vi "View.vi"(8 "error out":errorcluster, 11 "2-Axis Stage":refnum<class "2-Axis Stage Async API.lvclass">) -> (0 "error out":errorcluster)   [LabVIEW 2022 SP3, in "View.lvlib"]
uses:
  View.lvlib
  Interfaces/2-Axis Stage API/2-Axis Stage Async API.lvclass
panel:
  out "XY Position Graph":cluster{"X":dbl, "Y":dbl}[](graph)
  in  "Abort Motion":bool
  in  "Home Stage":bool
  in  "Move Stage":bool
  in  "Y-Destination":dbl
  in  "X-Destination":dbl
  in  "Clear Error":bool
  out "Y-Speed":dbl
  in  "Set Y-Speed":u16
  in  "Set Y-Acceleration":u16
  out "Y-Current Speed":dbl
  out "Y-Acceleration":dbl
  out "Y-Homed":bool
  out "Y-Moving":bool
  out "Y-Position":dbl
  out "X-Speed":dbl
  in  "Set X-Speed":u16
  in  "Set X-Acceleration":u16
  out "X-Current Speed":dbl
  out "X-Acceleration":dbl
  out "X-Homed":bool
  out "X-Moving":bool
  out "X-Position":dbl
  out "Stage Error":errorcluster
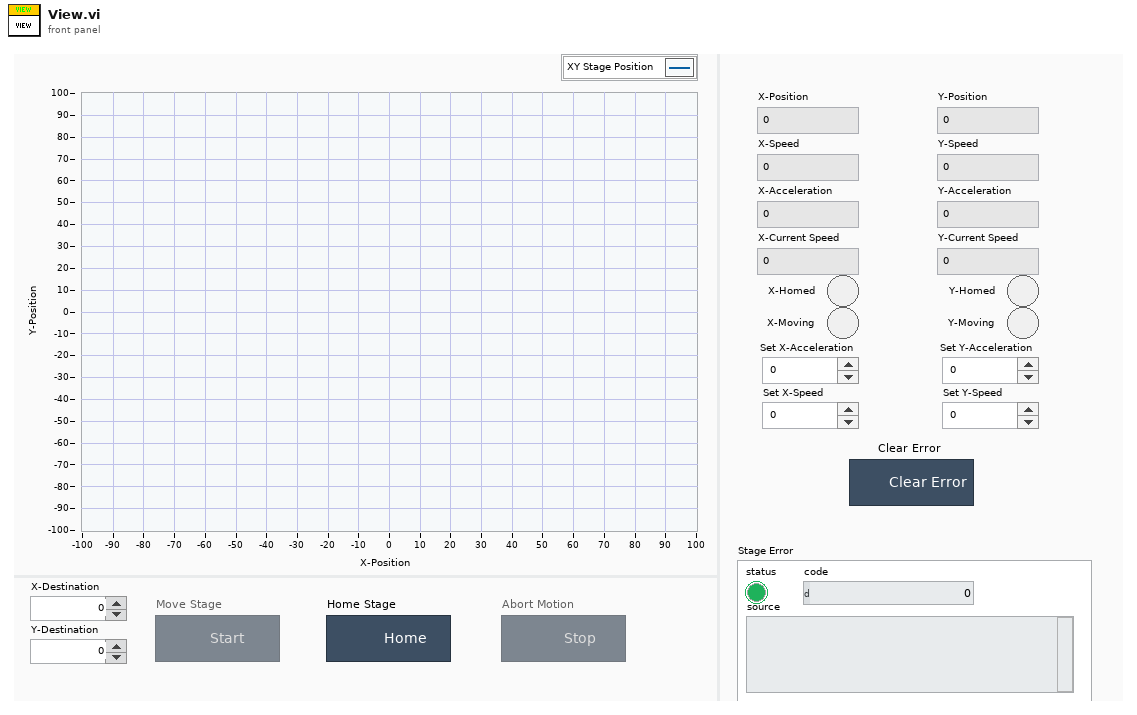
[diagram p1: front panel]
types:
  T1 = enum8{"Enabled", "Disabled", "Disabled and Grayed Out"}
  T2 = enum32{"Invalid", "Standard", "Closed", "Hidden", "Minimized", "Maximized"}
  T3 = enum32{"invalid app kind", "Development System", "Run Time System", "Student Edition", "Embedded LabVIEW", "Evaluation", "Custom"}
  T4 = cluster{"Current Position X":dbl, "Current Position Y":dbl}[]
  T5 = cluster{"Core":cluster{"Current VI Reference":refnum<vi>, "Close Panel on Exit?":bool}, "2-Axis Stage":refnum<class "2-Axis Stage Async API.lvclass">}
  T6 = cluster{"Current VI Reference":refnum<vi>, "Close Panel on Exit?":bool}
  T7 = cluster{"Event Registration Refnum":refnum<event-registration>, "Event Registration Refnum":refnum<event-registration>}
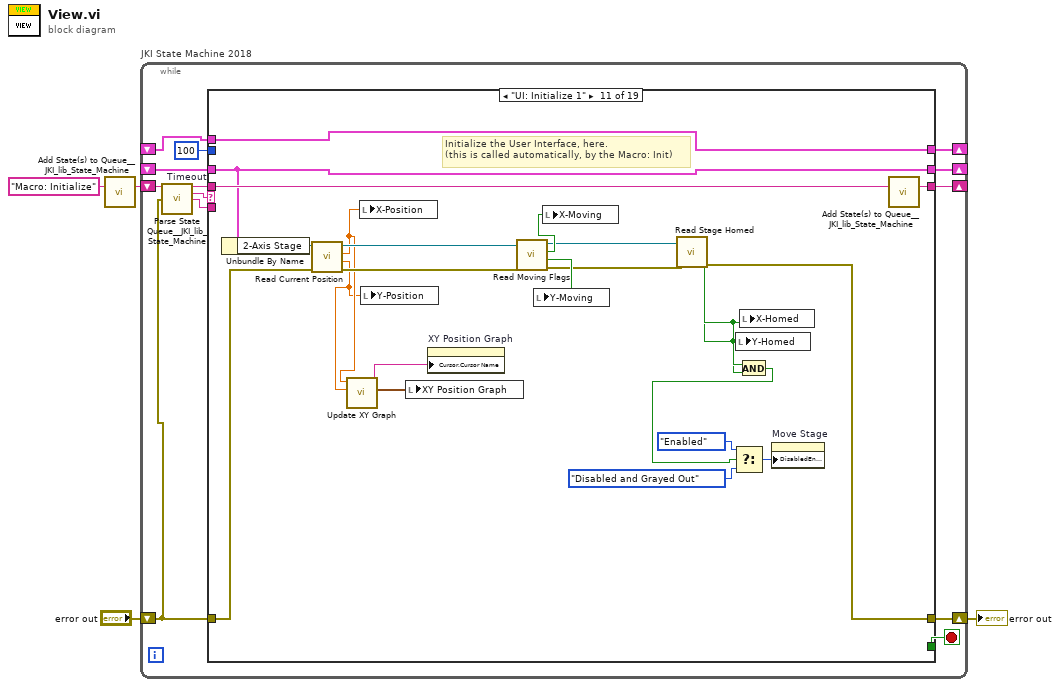
[diagram p0: block diagram]
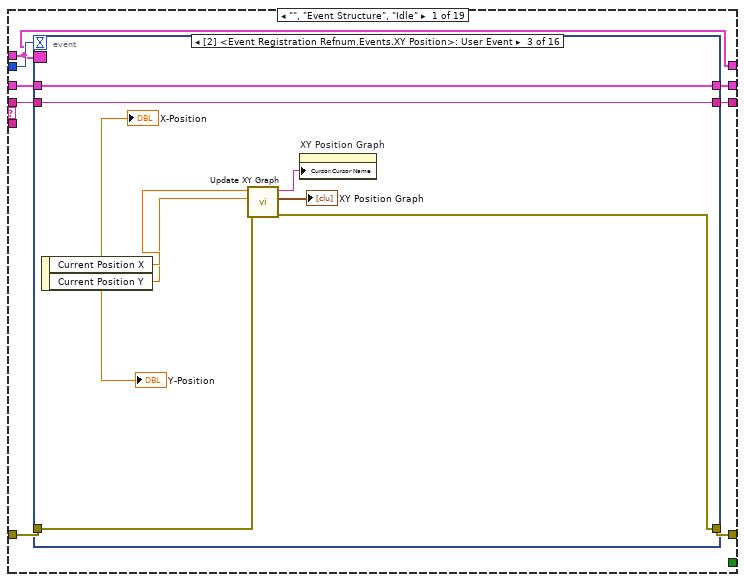
[diagram p2: hidden frame]
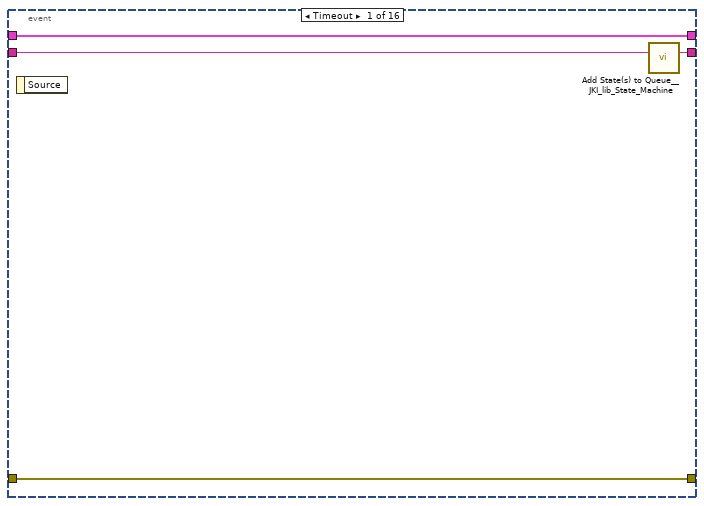
[diagram p3: hidden frame]
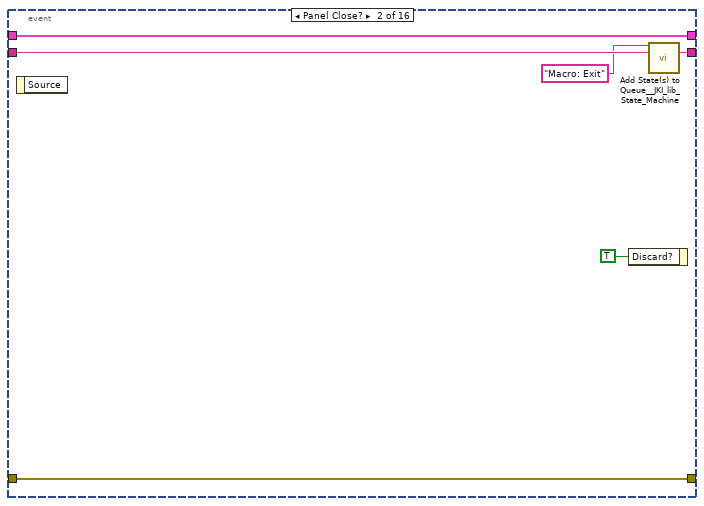
[diagram p4: hidden frame]
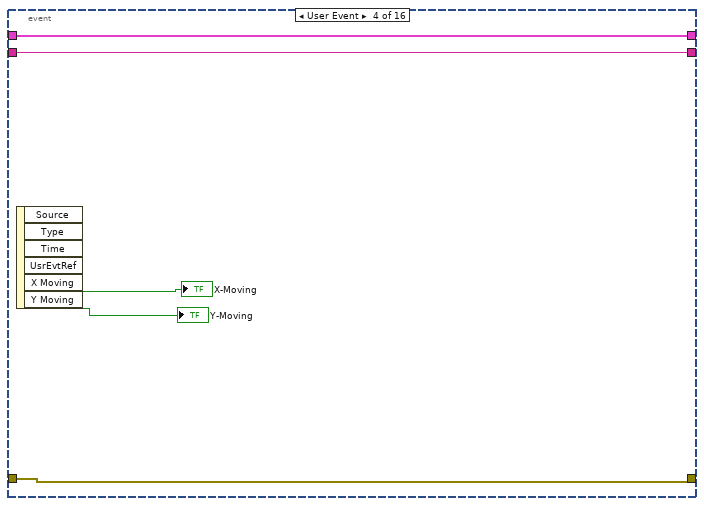
[diagram p5: hidden frame]
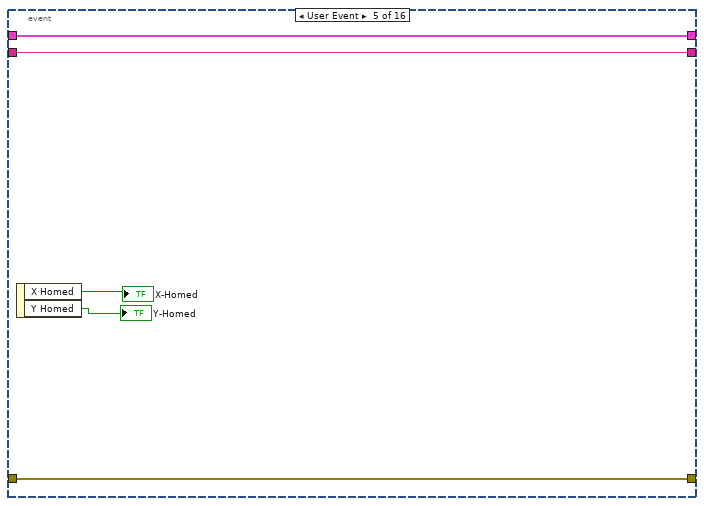
[diagram p6: hidden frame]
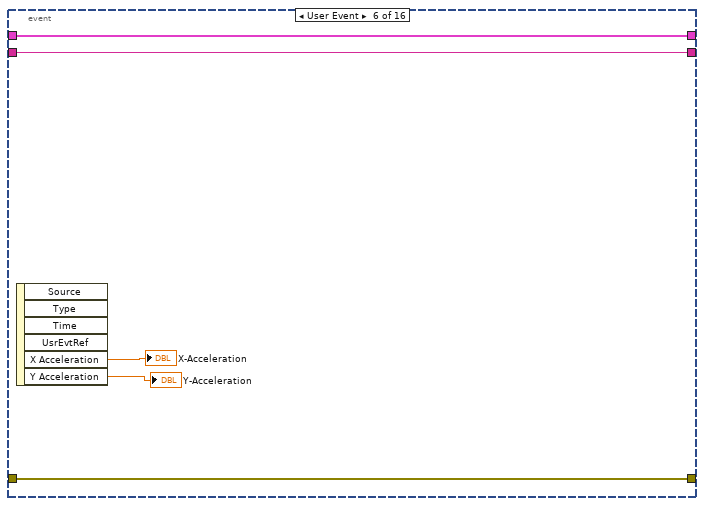
[diagram p7: hidden frame]
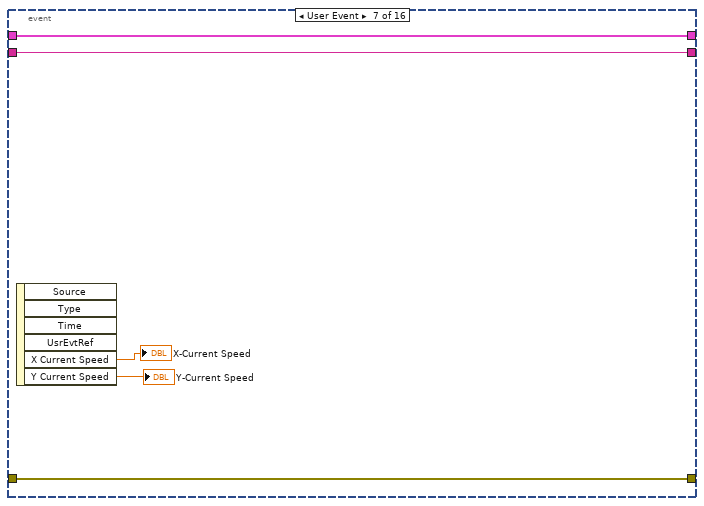
[diagram p8: hidden frame]
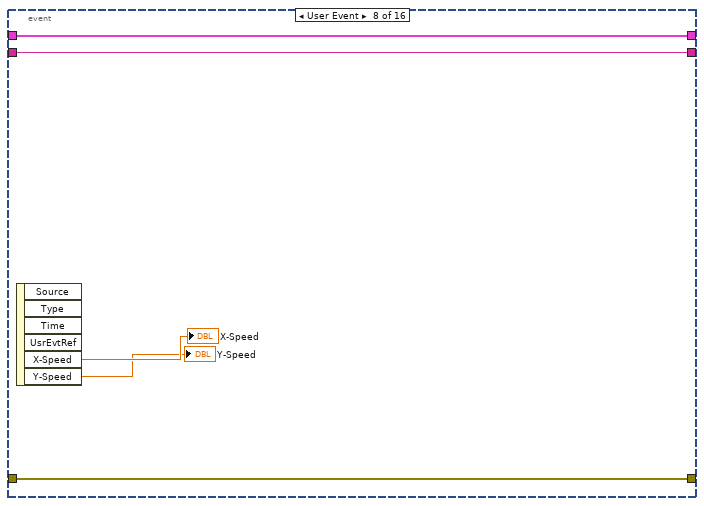
[diagram p9: hidden frame]
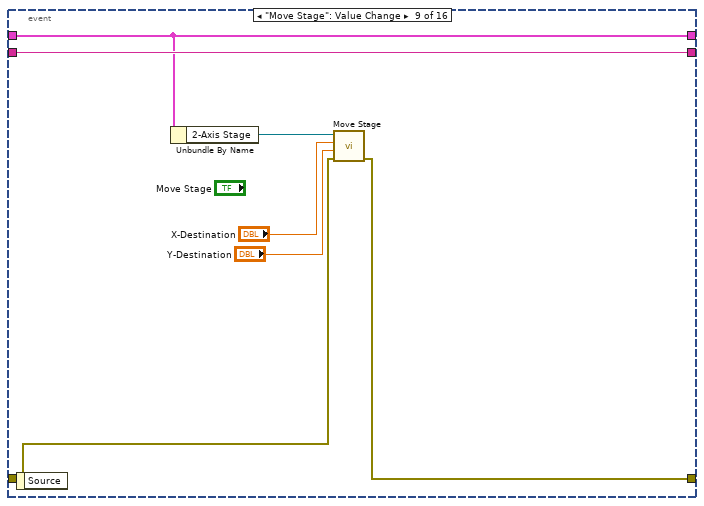
[diagram p10: hidden frame]
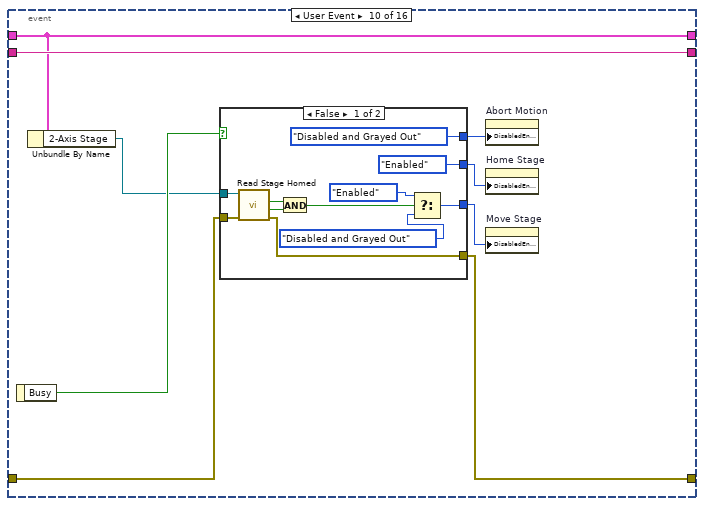
[diagram p11: hidden frame]
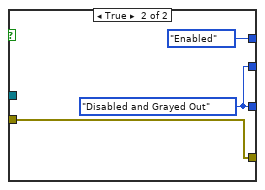
[diagram p12: hidden frame]
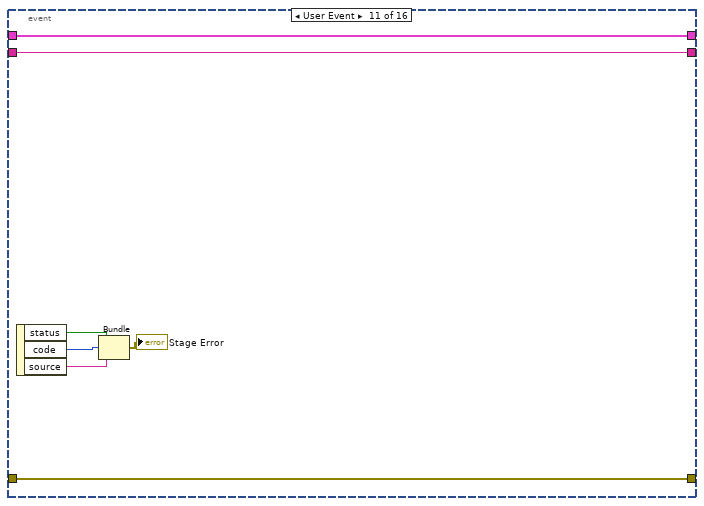
[diagram p13: hidden frame]
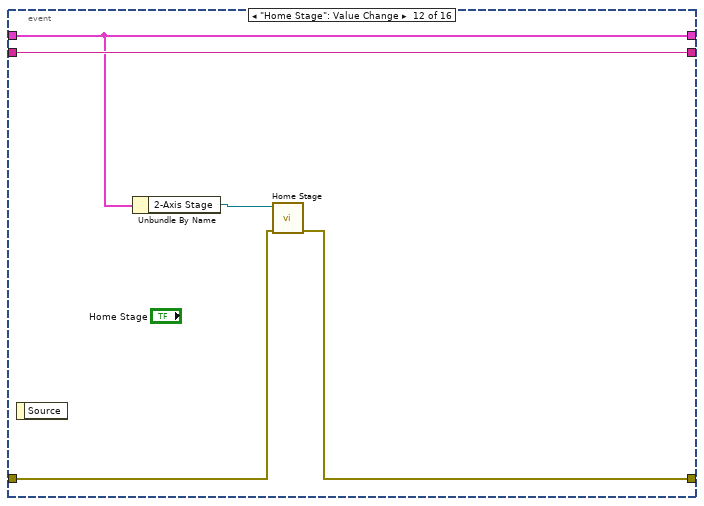
[diagram p14: hidden frame]
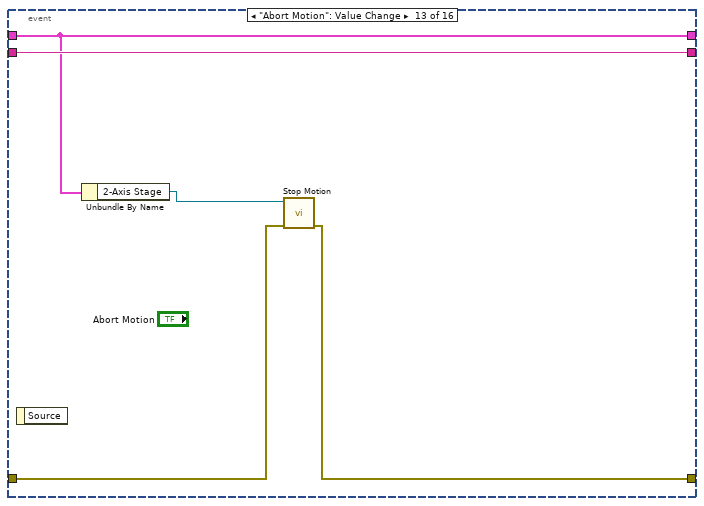
[diagram p15: hidden frame]
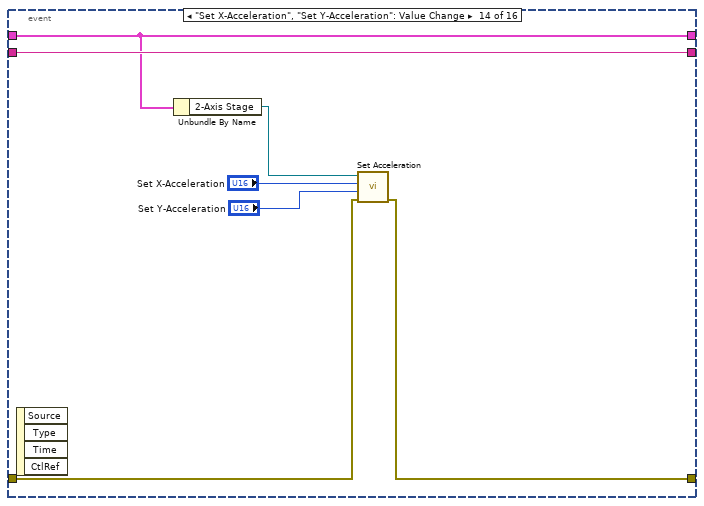
[diagram p16: hidden frame]
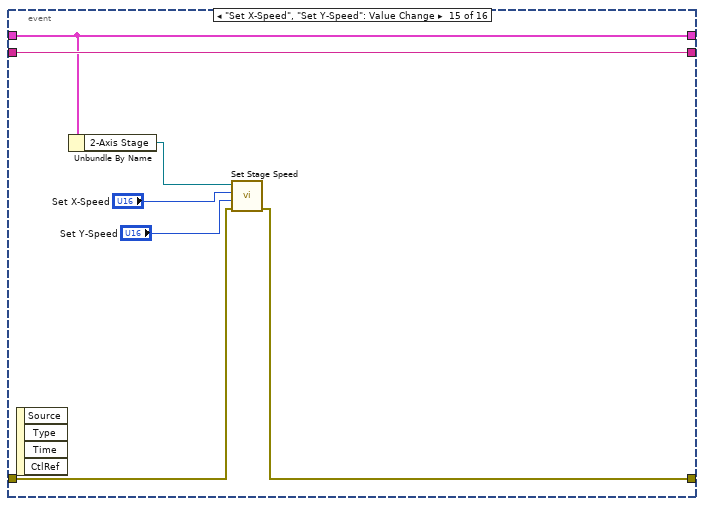
[diagram p17: hidden frame]
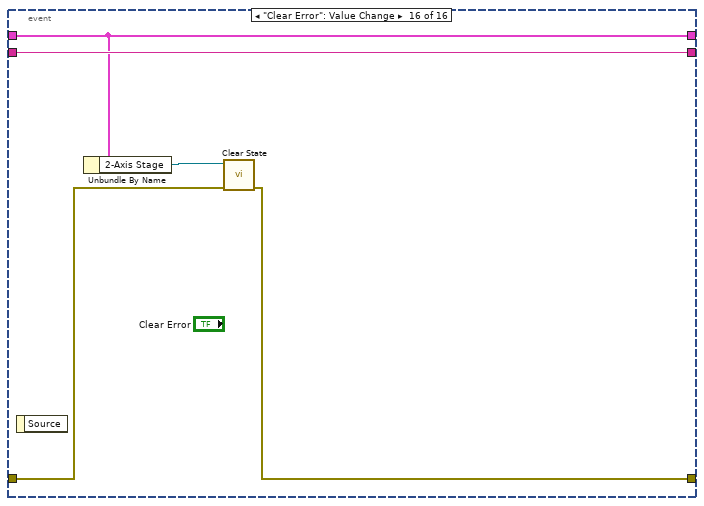
[diagram p18: hidden frame]
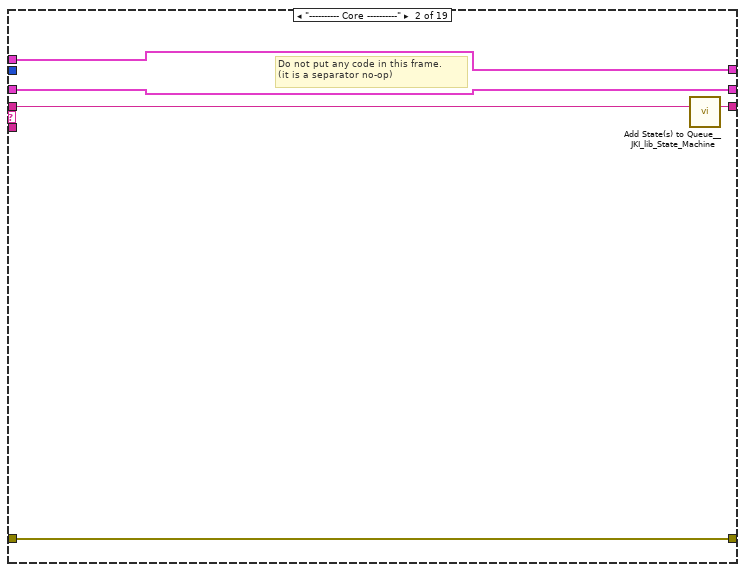
[diagram p19: hidden frame]
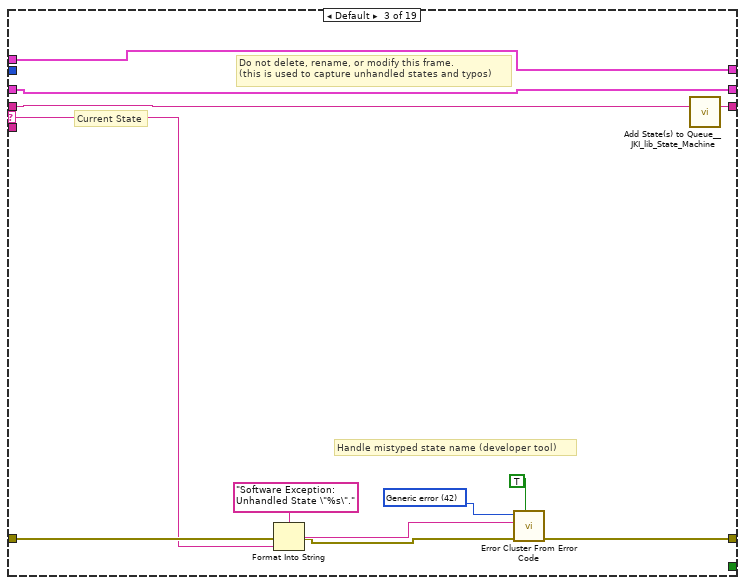
[diagram p20: hidden frame]
diagram:
  n1 = call <vilib>:"Add State(s) to Queue__JKI_lib_State_Machine.vi"("State(s) in (\"\")"="Macro: Initialize") -> ("States Out"=w4:string)  [unwired: 14 in]
  n2 = while "JKI State Machine 2018" {
    shift-right: [w10] -> _
    shift-left: _ -> [w9]
    shift-right: [w13] -> w1
    shift-left: "error out" -> [w7]
    shift-right: [w12] -> _
    shift-left: w4 -> [w14]
    shift-right: [w6] -> _
    shift-left: _ -> [w5]
    stop <- w11 stop-if-true
    w8 = 100  # Timeout
    n3 = call <vilib>:"Parse State Queue__JKI_lib_State_Machine.vi"("State Queue"=w14, "Error In (no error)"=w7) -> ("Remaining States"=w16:string, "Current State"=w17:string, "Arguments"=w15:string)  [unwired: 11 in]
    n4 = case shown="\"UI: Initialize 1\"" w17 {
      selector: w17 -> [_ _ w141 _ _ _ _ _ _ _ _ _ _ _ _ _ _ _ _]
      tunnel: w16 -> [w25 w139 w145 w165 w172 w178 w183 w190 w197 w202 w225 w241 w248 w260 w330 w336 w347 w352 w358]
      tunnel: w15 -> [_ _ _ _ _ _ _ _ _ _ _ _ w243 w254 _ _ _ _ _]
      tunnel: w9 -> [w23 w136 w143 w158 w169 w176 w180 _ w192 w199 w222 w229 w246 w256 w327 w333 w344 w349 w357]
      tunnel: [w22 w137 w147 w162 errorcluster {"status"=FALSE, "code"=0, "source"=""} ("error out") w175 w181 w187 w193 w200 w207 w226 w244 w257 w328 w334 w345 w350 w353] -> w13
      tunnel: w7 -> [w21 w137 w146 w162 w166 w175 w181 w187 w194 w200 w214 w227 w245 w258 w328 w334 w345 w350 w354]
      tunnel: [w24 w138 w144 w164 w171 w177 w182 w189 w196 w201 w224 w241 w247 w259 w329 w335 w346 w351 w358] -> w12
      tunnel: [_ _ _ _ _ TRUE _ _ _ _ _ _ _ _ _ _ _ _ _] -> w11
      tunnel: [w20 w136 w143 w163 w169 w176 w180 w188 w192 w199 w222 w229 w246 w256 w327 w333 w344 w349 w357] -> w10
      tunnel: w8 -> [w19 _ _ _ _ _ _ _ _ _ _ _ _ _ _ _ _ _ _]
      tunnel: [w18 w135 w140 w152 w167 w173 w179 w184 w191 w198 w223 w240 w242 w253 w326 w331 w337 w348 w355] -> w6
      tunnel: w5 -> [w18 w135 w140 w152 w167 w173 w179 w184 w191 w198 w223 w240 w242 w253 w326 w331 w337 w348 _]
      frame "", "Event Structure", "Idle" {
        n5 = event shown="[2] <Event Registration Refnum.Events.XY Position>: User Event" {
          selector: w18 -> [_ _ _ _ _ _ _ _ _ _ _ _ _ _ _ _]
          dyn-events: _ -> [_ _ _ _ _ _ _ _ _ _ _ _ _ _ _ _]
          timeout: w19 -> [_ _ _ _ _ _ _ _ _ _ _ _ _ _ _ _]
          tunnel: w25 -> [w29 w35 w42 w48 w53 w58 w63 w68 w75 w84 w105 w110 w115 w122 w129 w134]
          tunnel: [w28 w34 w42 w48 w53 w58 w63 w68 w75 w84 w105 w110 w115 w122 w129 w134] -> w24
          tunnel: w23 -> [w26 w32 w43 w47 w52 w57 w62 w67 w74 w80 w104 w109 w114 w121 w128 w133]
          tunnel: [w27 w33 w36 w44 w49 w54 w59 w64 w69 w76 w99 w106 w112 w116 w125 w130] -> w22
          tunnel: w21 -> [w27 w33 w37 w44 w49 w54 w59 w64 w70 w77 w99 w107 w111 w117 w126 w131]
          tunnel: [w26 w32 w43 w47 w52 w57 w62 w67 w74 w80 w104 w109 w114 w121 w128 w133] -> w20
          event Timeout {
            n6 = event-data() -> ()  [unwired: 1 in, 1 out]
            n7 = call <vilib>:"Add State(s) to Queue__JKI_lib_State_Machine.vi"("State(s) in (\"\")"=w29) -> ("States Out"=w28:string)  [unwired: 14 in]
          }
          event Panel Close? {
            n8 = event-data() -> ()  [unwired: 1 in, 1 out]
            n9 = event-data("Discard?"=TRUE) -> ()  [unwired: 1 in, 1 out]
            n10 = call <vilib>:"Add State(s) to Queue__JKI_lib_State_Machine.vi"("State(s) in Front (\"\")"="Macro: Exit", "State(s) in (\"\")"=w35) -> ("States Out"=w34:string)  [unwired: 13 in]
          }
          event User Event {
            n11 = event-data() -> ("Current Position X"=w40:dbl, "Current Position Y"=w39:dbl)  [unwired: 1 in]
            "Y-Position" <- w39
            "X-Position" <- w40
            n12 = call "Update XY Graph.vi"("error in (no error)"=w37, "Current Position Y"=w39, "Current Position X"=w40) -> ("error out"=w36:errorcluster, "Array"=→"XY Position Graph":T4, "String"=w38:string)  [unwired: 6 in]
            n13 = property on="XY Position Graph" class="XYGraph (strict)"("Cursor.Cursor Name"=w38) -> ()  [unwired: 2 in, 2 out]
          }
          event User Event {
            n14 = event-data() -> ("X Moving"=→"X-Moving":bool, "Y Moving"=→"Y-Moving":bool)  [unwired: 1 in, 4 out]
          }
          event User Event {
            n15 = event-data() -> ("X Homed"=→"X-Homed":bool, "Y Homed"=→"Y-Homed":bool)  [unwired: 1 in]
          }
          event User Event {
            n16 = event-data() -> ("X Acceleration"=→"X-Acceleration":dbl, "Y Acceleration"=→"Y-Acceleration":dbl)  [unwired: 1 in, 4 out]
          }
          event User Event {
            n17 = event-data() -> ("X Current Speed"=→"X-Current Speed":dbl, "Y Current Speed"=→"Y-Current Speed":dbl)  [unwired: 1 in, 4 out]
          }
          event User Event {
            n18 = event-data() -> ("X-Speed"=→"X-Speed":dbl, "Y-Speed"=→"Y-Speed":dbl)  [unwired: 1 in, 4 out]
          }
          event "Move Stage": Value Change {
            n19 = event-data() -> ()  [unwired: 1 in, 1 out]
            n20 = Unbundle By Name(w74) -> ("2-Axis Stage"=w73:refnum<class "2-Axis Stage Async API.lvclass">)
            n21 = call-dynamic "Move Stage.vi"("error in (no error)"=w70, "Y Axis"="Y-Destination", "X Axis"="X-Destination", "2-Axis Stage in"=w73) -> ("error out"=w69:errorcluster)  [unwired: 6 in, 1 out]
          }
          event User Event {
            n22 = event-data() -> ("Busy"=w83:bool)  [unwired: 1 in]
            n23 = Unbundle By Name(w80) -> ("2-Axis Stage"=w79:refnum<class "2-Axis Stage Async API.lvclass">)
            n24 = case shown="False" w83 {
              tunnel: [T1."Enabled" ("Disabled") w97] -> w82
              tunnel: [T1."Disabled and Grayed Out" ("Disabled") T1."Enabled" ("Disabled")] -> w81
              tunnel: w79 -> [w93 _]
              tunnel: [w87 w97] -> w78
              tunnel: w77 -> [w86 w96]
              tunnel: [w85 w96] -> w76
              frame False {
                n25 = call-dynamic "Read Stage Homed.vi"("error in (no error)"=w86, "2-Axis Stage Status in"=w93) -> ("error out"=w85:errorcluster, "Y-Axis Homed Moving"=w91:bool, "X-Axis Homed"=w92:bool)  [unwired: 6 in, 1 out]
                n26 = And(x=w92, y=w91) -> (x .and. y?=w90:bool)
                n27 = Select(t=T1."Enabled" ("Disabled"), s=w90, f=T1."Disabled and Grayed Out" ("Disabled")) -> (s? t:f=w87:T1)
              }
              frame True {
                w97 = T1."Disabled and Grayed Out" ("Disabled")
              }
            }
            n28 = property on="Abort Motion" class="Bool"("DisabledEnum"=w81) -> ()  [unwired: 2 in, 2 out]
            n29 = property on="Home Stage" class="Bool"("DisabledEnum"=w82) -> ()  [unwired: 2 in, 2 out]
            n30 = property on="Move Stage" class="Bool"("DisabledEnum"=w78) -> ()  [unwired: 2 in, 2 out]
          }
          event User Event {
            n31 = event-data() -> ("status"=w103:bool, "code"=w102:i32, "source"=w101:string)  [unwired: 1 in]
            n32 = Bundle("status"=w103, "code"=w102, "source"=w101) -> (→"Stage Error":errorcluster)  [unwired: 1 in]
          }
          event "Home Stage": Value Change {
            n33 = event-data() -> ()  [unwired: 1 in, 1 out]
            n34 = Unbundle By Name(w109) -> ("2-Axis Stage"=w108:refnum<class "2-Axis Stage Async API.lvclass">)
            n35 = call-dynamic "Home Stage.vi"("error in (no error)"=w107, "2-Axis Stage in"=w108) -> ("error out"=w106:errorcluster)  [unwired: 8 in, 1 out]
          }
          event "Abort Motion": Value Change {
            n36 = event-data() -> ()  [unwired: 1 in, 1 out]
            n37 = Unbundle By Name(w114) -> ("2-Axis Stage"=w113:refnum<class "2-Axis Stage Async API.lvclass">)
            n38 = call-dynamic "Stop Motion.vi"("error in (no error)"=w111, "2-Axis Stage in"=w113) -> ("error out"=w112:errorcluster)  [unwired: 8 in, 1 out]
          }
          event "Set X-Acceleration", "Set Y-Acceleration": Value Change {
            n39 = event-data() -> ()  [unwired: 1 in, 4 out]
            n40 = Unbundle By Name(w121) -> ("2-Axis Stage"=w120:refnum<class "2-Axis Stage Async API.lvclass">)
            n41 = call-dynamic "Set Acceleration.vi"("error in (no error)"=w117, "Y Axis"="Set Y-Acceleration", "X Axis"="Set X-Acceleration", "2-Axis Stage in"=w120) -> ("error out"=w116:errorcluster)  [unwired: 6 in, 1 out]
          }
          event "Set X-Speed", "Set Y-Speed": Value Change {
            n42 = event-data() -> ()  [unwired: 1 in, 4 out]
            n43 = Unbundle By Name(w128) -> ("2-Axis Stage"=w127:refnum<class "2-Axis Stage Async API.lvclass">)
            n44 = call-dynamic "Set Stage Speed.vi"("error in (no error)"=w126, "Y Axis"="Set Y-Speed", "X Axis"="Set X-Speed", "2-Axis Stage in"=w127) -> ("error out"=w125:errorcluster)  [unwired: 6 in, 1 out]
          }
          event "Clear Error": Value Change {
            n45 = event-data() -> ()  [unwired: 1 in, 1 out]
            n46 = Unbundle By Name(w133) -> ("2-Axis Stage"=w132:refnum<class "2-Axis Stage Async API.lvclass">)
            n47 = call-dynamic "Clear State.vi"("error in (no error)"=w131, "2-Axis Stage Status in"=w132) -> ("error out"=w130:errorcluster)  [unwired: 8 in, 1 out]
          }
        }
      }
      frame "---------- Core ----------" {
        # "Do not put any code in this frame.\n(it is a separator no-op)"
        n48 = call <vilib>:"Add State(s) to Queue__JKI_lib_State_Machine.vi"("State(s) in (\"\")"=w139) -> ("States Out"=w138:string)  [unwired: 14 in]
      }
      frame Default {
        w150 = 42 items=["No error", "Argument error", "Memory is full", "Out of zone", "End of file", "File already open", "Generic file I/O error", "File not found", "File permission error", "Disk is full", "Duplicate path", "Too many files open", "System feature not enabled", "Resource file not found", "Cannot add resource", "Resource not found", "Image not found", "Image memory error", "Pen does not exist", "Config type invalid", "Config token not found", "Config parse error", "Config memory error", "Bad external code format", "Bad external code offset", "External code not present", "Null window", "Destroy window error", "Null menu", "Print aborted", "Bad print record", "Print driver error", "Windows error during printing", "Memory error during printing", "Print dialog error", "Generic print error", "Invalid device refnum", "Device not found", "Device parameter error", "Device unit error", "Cannot open device", "Device call aborted", "Generic error", "Cancelled by user", "Object ID too low", "Object ID too high", "Object not in heap", "Unknown heap", "Unknown object (invalid DefProc)", "Unknown object (DefProc not in table)", "Message out of range", "Invalid (null) method", "Unknown message", "Manager call not supported", "Bad address", "Network operation in progress", "Network operation timed out", "Connection is busy", "Network attribute not supported", "Network error", "Address in use", "System out of memory", "Connection aborted", "Connection refused", "Not connected", "Already connected", "Connection closed", "Initialization error (interapplication manager)", "Bad occurrence", "Wait on unbound occurrence handler", "Occurrence queue overflow", "Datalog type conflict", "Unused", "Unrecognized type (interapplication manager)", "Memory corrupt", "Failed to make temporary DLL", "Old CIN version", "Drag socket not found", "Failed to load drop-object", "Failed to register OLE object", "Failed to release OLE object", "Format specifier type mismatch", "Unknown format specifier", "Too few format specifiers", "Too many format specifiers", "Scan failed", "Newer CIN version", "Error converting to variant", "Runtime menu error", "Password tampered", "Variant attribute not found", "Incompatible variant data type", "Event data is not available", "Event Store is not present", "Occurrence is not found", "Event Queue is not created", "Event info is not available", "Refnum passed is NULL", "Error retrieving Class GUID", "Error retrieving CoClass GUID", "Error retrieving TypeLib GUID.", "Bad built application magic bytes.", "Specific driver is different from the specific driver associated with the Logical Name.", "There is no session opened to the class driver.", "Max Error", "MAX - Error with config objects", "MAX - Error loading configuration", "MAX - Group not supported"]
        # "Current State"
        # "Do not delete, rename, or modify this frame.\n(this is used to capture unhandled states and typos)"
        # "Handle mistyped state name (developer tool)"
        n49 = Format Into String(format string="Software Exception: Unhandled State \"%s\"." ("message"), error in=w146, w141) -> (resulting string=w149:string, error out=w148:errorcluster)  [unwired: 1 in]
        n50 = call <vilib>:"Error Cluster From Error Code.vi"("show call chain? (False)"=TRUE, "error in (no error)"=w148, "error message (\"\")"=w149, "error code (0)"=w150) -> ("error out"=w147:errorcluster)  [unwired: 5 in]
        n51 = call <vilib>:"Add State(s) to Queue__JKI_lib_State_Machine.vi"("State(s) in (\"\")"=w145) -> ("States Out"=w144:string)  [unwired: 14 in]
      }
      frame "Initialize Core Data" {
        # "Do not delete, rename, or modify this frame.\n(this is used to determine panel behavior on exit)"
        # "originally closed?"
        # "exe?"
        # "If panel starts closed or is an EXE, then close it when we exit"
        n52 = property class="VI"() -> ("FP.State"=w155:T2)  [unwired: 2 in, 2 out]
        n53 = property class="App"() -> ("App.Kind"=w161:T3)  [unwired: 2 in, 2 out]
        n54 = control-ref of="Current VI Reference"() -> (w156:refnum<vi>)
        n55 = Equal?(x=w155, y=T2."Closed" ("Front Panel Window:State")) -> (x = y?=w153:bool)
        n56 = Equal?(x=w161, y=T3."Run Time System" ("Application:Kind")) -> (x = y?=w159:bool)
        n57 = Or(x=w153, y=w159) -> (x .or. y?=w157:bool)
        n58 = Bundle By Name(cluster=w158, "Core.Current VI Reference"=w156, "Core.Close Panel on Exit?"=w157) -> (w163:T5)
        n59 = call <vilib>:"Add State(s) to Queue__JKI_lib_State_Machine.vi"("State(s) in (\"\")"=w165) -> ("States Out"=w164:string)  [unwired: 14 in]
      }
      frame "Error Handler" {
        # "Handle any errors here.\nYou can also output any states to clean-up after errors occur"
        # "Clear error"
        n60 = local write "Stage Error"(w166) -> ()
        n61 = call <vilib>:"Add State(s) to Queue__JKI_lib_State_Machine.vi"("State(s) in Front (\"\")"="/* Post Error States", "State(s) in (\"\")"=w172) -> ("States Out"=w171:string)  [unwired: 13 in]
      }
      frame "Exit" {
        # "Do not put any code in this frame.\n(No errors that occur here will be handled.)"
        n62 = call <vilib>:"Add State(s) to Queue__JKI_lib_State_Machine.vi"("State(s) in (\"\")"=w178) -> ("States Out"=w177:string)  [unwired: 14 in]
      }
      frame "---------- Data ----------" {
        # "Do not put any code in this frame.\n(It is a separator no-op. You can make a copy of this frame to create a new Data frame)"
        n63 = call <vilib>:"Add State(s) to Queue__JKI_lib_State_Machine.vi"("State(s) in (\"\")"=w183) -> ("States Out"=w182:string)  [unwired: 14 in]
      }
      frame "Data: Initialize" {
        w186 = T6 {"Current VI Reference"=refnum, "Close Panel on Exit?"=FALSE}  # Core
        # "Data names and types of shift register data are defined by this bundle."
        # "Initialize the shift-register data, here.\n(data names are defined by what you wire into the bundle function)"
        n64 = Bundle("Core"=w186, "2-Axis Stage"="2-Axis Stage") -> (w188:T5)  [unwired: 1 in]
        n65 = call <vilib>:"Add State(s) to Queue__JKI_lib_State_Machine.vi"("State(s) in (\"\")"=w190) -> ("States Out"=w189:string)  [unwired: 14 in]
      }
      frame "Data: Cleanup" {
        # "Cleanup any data and references, here.\n(this is called automatically, by the Macro: Exit)"
        n66 = Unbundle By Name(w192) -> ("Core.Current VI Reference"=w195:refnum<vi>)
        n67 = Close Reference(reference=w195, error in (no error)=w194) -> (error out=w193:errorcluster)
        n68 = call <vilib>:"Add State(s) to Queue__JKI_lib_State_Machine.vi"("State(s) in (\"\")"=w197) -> ("States Out"=w196:string)  [unwired: 14 in]
      }
      frame "---------- UI ----------" {
        # "Do not put any code in this frame.\n(It is a separator no-op. You can make a copy of this frame to create a new UI frame)"
        n69 = call <vilib>:"Add State(s) to Queue__JKI_lib_State_Machine.vi"("State(s) in (\"\")"=w202) -> ("States Out"=w201:string)  [unwired: 14 in]
      }
      frame "UI: Initialize 1" {
        # "Initialize the User Interface, here.\n(this is called automatically, by the Macro: Init)"
        n70 = Unbundle By Name(w222) -> ("2-Axis Stage"=w219:refnum<class "2-Axis Stage Async API.lvclass">)
        n71 = call-dynamic "Read Current Position.vi"("error in (no error)"=w214, "2-Axis Stage Status in"=w219) -> ("error out"=w216:errorcluster, "Y Position"=w205:dbl, "X Position"=w206:dbl, "2-Axis Stage Status out"=w218:refnum<class "2-Axis Stage Async API.lvclass">)  [unwired: 6 in]
        n72 = call "Update XY Graph.vi"("Current Position Y"=w205, "Current Position X"=w206) -> ("Array"=w204:T4, "String"=w203:string)  [unwired: 7 in, 1 out]
        n73 = local write "X-Position"(w206) -> ()
        n74 = local write "Y-Position"(w205) -> ()
        n75 = local write "XY Position Graph"(w204) -> ()
        n76 = property on="XY Position Graph" class="XYGraph (strict)"("Cursor.Cursor Name"=w203) -> ()  [unwired: 2 in, 2 out]
        n77 = call-dynamic "Read Moving Flags.vi"("error in (no error)"=w216, "2-Axis Stage Status in"=w218) -> ("error out"=w215:errorcluster, "Y-Axis Moving"=w220:bool, "X-Axis Moving"=w221:bool, "2-Axis Stage Status out"=w217:refnum<class "2-Axis Stage Async API.lvclass">)  [unwired: 6 in]
        n78 = local write "Y-Moving"(w220) -> ()
        n79 = local write "X-Moving"(w221) -> ()
        n80 = call-dynamic "Read Stage Homed.vi"("error in (no error)"=w215, "2-Axis Stage Status in"=w217) -> ("error out"=w207:errorcluster, "Y-Axis Homed Moving"=w212:bool, "X-Axis Homed"=w213:bool)  [unwired: 6 in, 1 out]
        n81 = local write "Y-Homed"(w212) -> ()
        n82 = And(x=w213, y=w212) -> (x .and. y?=w211:bool)
        n83 = Select(t=T1."Enabled" ("Disabled"), s=w211, f=T1."Disabled and Grayed Out" ("Disabled")) -> (s? t:f=w209:T1)
        n84 = local write "X-Homed"(w213) -> ()
        n85 = property on="Move Stage" class="Bool"("DisabledEnum"=w209) -> ()  [unwired: 2 in, 2 out]
        n86 = call <vilib>:"Add State(s) to Queue__JKI_lib_State_Machine.vi"("State(s) in (\"\")"=w225) -> ("States Out"=w224:string)  [unwired: 14 in]
      }
      frame "UI: Initialize 2" {
        n87 = Unbundle By Name(w229) -> ("2-Axis Stage"=w228:refnum<class "2-Axis Stage Async API.lvclass">)
        n88 = call-dynamic "Read Current Speed.vi"("error in (no error)"=w227, "2-Axis Stage Status in"=w228) -> ("error out"=w236:errorcluster, "Y Current Speed"=w239:dbl, "X Current Speed"=w238:dbl, "2-Axis Stage Status out"=w237:refnum<class "2-Axis Stage Async API.lvclass">)  [unwired: 6 in]
        n89 = local write "X-Current Speed"(w238) -> ()
        n90 = local write "Y-Current Speed"(w239) -> ()
        n91 = call-dynamic "Read Acceleration.vi"("error in (no error)"=w236, "2-Axis Stage Status in"=w237) -> ("error out"=w234:errorcluster, "Y Acceleration"=w230:dbl, "X Acceleration"=w231:dbl, "2-Axis Stage Status out"=w235:refnum<class "2-Axis Stage Async API.lvclass">)  [unwired: 6 in]
        n92 = local write "Set Y-Acceleration"(w230) -> ()
        n93 = local write "Y-Acceleration"(w230) -> ()
        n94 = local write "X-Acceleration"(w231) -> ()
        n95 = local write "Set X-Acceleration"(w231) -> ()
        n96 = call-dynamic "Read Speed.vi"("error in (no error)"=w234, "2-Axis Stage Status in"=w235) -> ("error out"=w226:errorcluster, "Y-Axis Speed"=w232:dbl, "X-Axis Speed"=w233:dbl)  [unwired: 6 in, 1 out]
        n97 = local write "Set X-Speed"(w233) -> ()
        n98 = local write "X-Speed"(w233) -> ()
        n99 = local write "Y-Speed"(w232) -> ()
        n100 = local write "Set Y-Speed"(w232) -> ()
      }
      frame "UI: Cursor Set" {
        # "Argument"
        # "Set and Unset Cursor Busy.\n(Usage: \"UI: Cursor Set >> Busy|Idle\")"
        n101 = case shown="\"Idle\", Default" w243 {
          tunnel: w245 -> [w250 w252]
          tunnel: [w249 w251] -> w244
          frame "Idle", Default {
            n102 = call <vilib>:"Unset Busy.vi"("error in (no error)"=w250) -> ("error out"=w249:errorcluster)  [unwired: 10 in]
          }
          frame "Busy" {
            n103 = call <vilib>:"Set Busy.vi"("error in (no error)"=w252) -> ("error out"=w251:errorcluster)  [unwired: 9 in, 1 out]
          }
        }
        n104 = call <vilib>:"Add State(s) to Queue__JKI_lib_State_Machine.vi"("State(s) in (\"\")"=w248) -> ("States Out"=w247:string)  [unwired: 14 in]
      }
      frame "UI: Front Panel State" {
        # "Argument"
        # "Set Front Panel Open or Closed\n(Usage: \"UI: Front Panel State >> Open|Close\")"
        n105 = Unbundle By Name(w256) -> ("Core.Current VI Reference"=w255:refnum<vi>)
        n106 = case shown="\"Minimize\", \"Minimized\"" w254 {
          tunnel: w258 -> [w266 w281 w292 w305 w318]
          tunnel: [w268 w282 w294 w307 w320] -> w257
          tunnel: w255 -> [w267 w279 w293 w306 w319]
          frame "Open", "Standard", Default {
            w261 = T2."Standard" ("State")
            n107 = property class="VI"(reference=w267, error in=w266) -> (reference out=w264:refnum<vi>, error out=w265:errorcluster, "FP.State"=w263:T2)
            n108 = Not Equal?(x=w263, y=w261) -> (x != y?=w262:bool)
            n109 = case shown="True" w262 {
              tunnel: [w272 w274] -> w268
              tunnel: w265 -> [w271 w274]
              tunnel: w264 -> [w270 _]
              tunnel: w261 -> [w269 _]
              frame True {
                n110 = invoke class="VI" method="FP.Open"(reference=w270, error in=w271, "Activate"=TRUE, "State"=w269) -> (error out=w272:errorcluster)  [unwired: 1 in, 4 out]
              }
              frame False {
              }
            }
          }
          frame "Close", "Closed" {
            n111 = property class="VI"(reference=w279, error in=w281) -> (reference out=w278:refnum<vi>, error out=w280:errorcluster, "FP.State"=w276:T2)
            n112 = Not Equal?(x=w276, y=T2."Closed" ("Front Panel Window:State")) -> (x != y?=w275:bool)
            n113 = case shown="True" w275 {
              tunnel: [w283 w286] -> w282
              tunnel: w280 -> [w283 w285]
              tunnel: w278 -> [_ w284]
              frame False {
              }
              frame True {
                n114 = invoke class="VI" method="FP.Close"(reference=w284, error in=w285) -> (error out=w286:errorcluster)  [unwired: 1 in, 2 out]
              }
            }
          }
          frame "Hidden", "Hide" {
            w287 = T2."Hidden" ("State")
            n115 = property class="VI"(reference=w293, error in=w292) -> (reference out=w290:refnum<vi>, error out=w291:errorcluster, "FP.State"=w289:T2)
            n116 = Not Equal?(x=w289, y=w287) -> (x != y?=w288:bool)
            n117 = case shown="True" w288 {
              tunnel: [w298 w299] -> w294
              tunnel: w291 -> [w297 w299]
              tunnel: w290 -> [w296 _]
              tunnel: w287 -> [w295 _]
              frame True {
                n118 = invoke class="VI" method="FP.Open"(reference=w296, error in=w297, "State"=w295) -> (error out=w298:errorcluster)  [unwired: 2 in, 4 out]
              }
              frame False {
              }
            }
          }
          frame "Minimize", "Minimized" {
            w300 = T2."Minimized" ("State")
            n119 = property class="VI"(reference=w306, error in=w305) -> (reference out=w303:refnum<vi>, error out=w304:errorcluster, "FP.State"=w302:T2)
            n120 = Not Equal?(x=w302, y=w300) -> (x != y?=w301:bool)
            n121 = case shown="True" w301 {
              tunnel: [w311 w312] -> w307
              tunnel: w304 -> [w310 w312]
              tunnel: w303 -> [w309 _]
              tunnel: w300 -> [w308 _]
              frame True {
                n122 = invoke class="VI" method="FP.Open"(reference=w309, error in=w310, "State"=w308) -> (error out=w311:errorcluster)  [unwired: 2 in, 4 out]
              }
              frame False {
              }
            }
          }
          frame "Maximize", "Maximized" {
            w313 = T2."Maximized" ("State")
            n123 = property class="VI"(reference=w319, error in=w318) -> (reference out=w316:refnum<vi>, error out=w317:errorcluster, "FP.State"=w315:T2)
            n124 = Not Equal?(x=w315, y=w313) -> (x != y?=w314:bool)
            n125 = case shown="True" w314 {
              tunnel: [w324 w325] -> w320
              tunnel: w317 -> [w323 w325]
              tunnel: w316 -> [w322 _]
              tunnel: w313 -> [w321 _]
              frame True {
                n126 = invoke class="VI" method="FP.Open"(reference=w322, error in=w323, "State"=w321) -> (error out=w324:errorcluster)  [unwired: 2 in, 4 out]
              }
              frame False {
              }
            }
          }
        }
        n127 = call <vilib>:"Add State(s) to Queue__JKI_lib_State_Machine.vi"("State(s) in (\"\")"=w260) -> ("States Out"=w259:string)  [unwired: 14 in]
      }
      frame "---------- Macro ----------" {
        # "Do not put any code in this frame.\n(It is a separator no-op. You can make a copy of this frame to create a new Macro frame)"
        n128 = call <vilib>:"Add State(s) to Queue__JKI_lib_State_Machine.vi"("State(s) in (\"\")"=w330) -> ("States Out"=w329:string)  [unwired: 14 in]
      }
      frame "Macro: Initialize" {
        w332 = "Data: Initialize\nInitialize Core Data\nEvents: Register for Events\nUI: Initialize 1\nUI: Initialize 2\nUI: Front Panel State >> Open"  # Data: Initialize Initialize Core Data Events: Register for Events UI: Initialize 1 UI: Initialize 2 UI: Front Panel State >> Open
        # "Initialization Macro\n(This is called once, when the VI starts)"
        n129 = call <vilib>:"Add State(s) to Queue__JKI_lib_State_Machine.vi"("State(s) in Front (\"\")"=w332, "State(s) in (\"\")"=w336) -> ("States Out"=w335:string)  [unwired: 13 in]
      }
      frame "Macro: Exit" {
        # "Exit Macro\n(This is called once, when the VI exits)"
        n130 = Unbundle By Name(w344) -> ("Core.Close Panel on Exit?"=w343:bool)
        n131 = Select(t="UI: Front Panel State >> Close", s=w343, f="") -> (s? t:f=w340:string)
        n132 = call <vilib>:"Add State(s) to Queue__JKI_lib_State_Machine.vi"("State(s) in (\"\")"=w340, "State(s) at Back (\"\")"="Data: Cleanup\nExit") -> ("States Out"=w338:string)  [unwired: 13 in]
        n133 = call <vilib>:"Add State(s) to Queue__JKI_lib_State_Machine.vi"("State(s) in Front (\"\")"=w338, "State(s) in (\"\")"=w347) -> ("States Out"=w346:string)  [unwired: 13 in]
      }
      frame "---------- Events ----------" {
        # "Template Separator\n(You can make a copy of, or modify, this frame)"
        n134 = call <vilib>:"Add State(s) to Queue__JKI_lib_State_Machine.vi"("State(s) in (\"\")"=w352) -> ("States Out"=w351:string)  [unwired: 14 in]
      }
      frame "Events: Register for Events" {
        n135 = Unbundle By Name(w357) -> ("2-Axis Stage"=w356:refnum<class "2-Axis Stage Async API.lvclass">)
        n136 = call-dynamic "Register for Events.vi"("error in (no error)"=w354, "Async Coms in"=w356) -> ("error out"=w353:errorcluster, "Event Refnums"=w355:T7)  [unwired: 7 in, 1 out]
      }
    }
  }
  "error out" <- w1
